vi "Set Power Off Ref.vi"(8 "error in (no error)":errorcluster, 10 "Self Test":refnum<vi>, 11 "Device Under Test In":refnum<class "Device Under Test.lvclass">) -> (0 "error out":errorcluster, 3 "Device Under Test Out":refnum<class "Device Under Test.lvclass">)   [LabVIEW 2021, in "Device Under Test.lvclass"]
uses:
  Device Under Test.lvclass
  C:/Program Files (x86)/National Instruments/LabVIEW 2021/vi.lib/Astemes/Triarc Framework/Process/Process.lvclass
  <vilib>/Astemes/Triarc Framework/Process/Process.lvclass/Process.ctl
  Device Under Test.lvclass/Device Under Test.ctl
  <vilib>/Utility/error.llb/Clear Errors.vi
  <vilib>/Astemes/Triarc Framework/Process/Private/SubVIs/Handle Debug Data.vi
  <vilib>/Utility/High Resolution Relative Seconds.vi
  <vilib>/Utility/error.llb/Error Cluster From Error Code.vi
  <vilib>/Astemes/Triarc Framework/Process/Process.lvclass
  C:/Program Files (x86)/National Instruments/LabVIEW 2021/vi.lib/Astemes/Triarc Framework/View/View.lvclass
  C:/Program Files (x86)/National Instruments/LabVIEW 2021/vi.lib/Astemes/Triarc Framework/Base/Base.lvclass
  C:/Program Files (x86)/National Instruments/LabVIEW 2021/vi.lib/Astemes/Triarc Framework/Error Handler Interface/Error Handler Interface.lvclass
  C:/Program Files (x86)/National Instruments/LabVIEW 2021/vi.lib/Astemes/Triarc Framework/Logging/Logging.lvclass
  C:/Git/astemes-triarc-examples/Thermal Chamber/Device Under Test/Device Under Test.lvclass
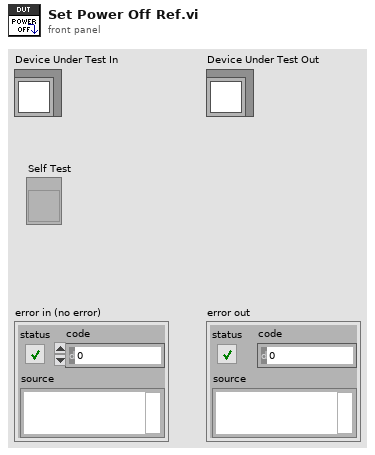
[diagram p1: front panel]
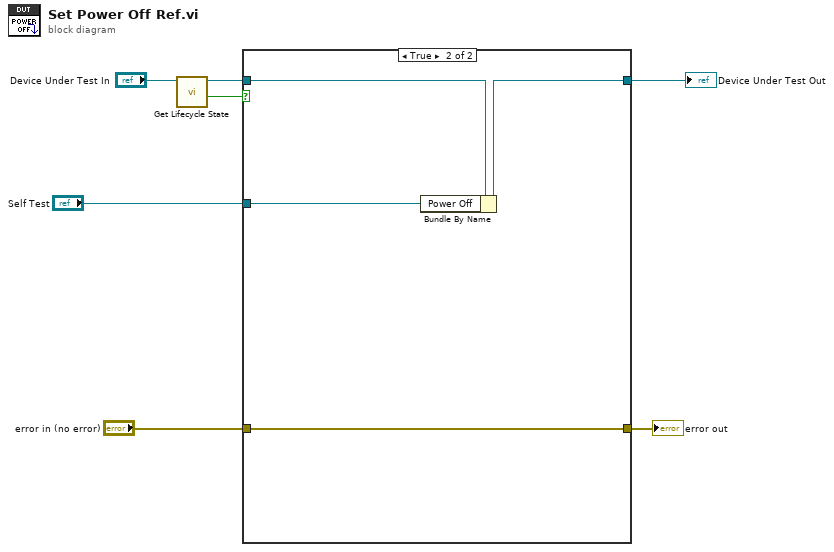
[diagram p0: block diagram]
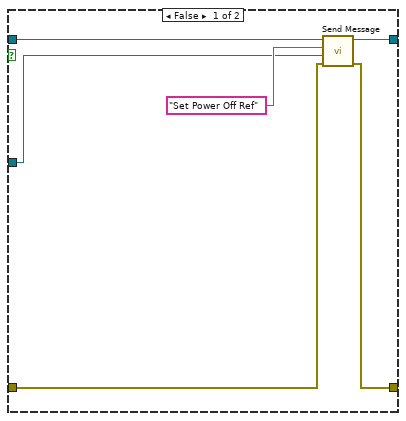
[diagram p2: hidden frame]
diagram:
  n1 = call <vilib>:"Get Lifecycle State.vi"("Process In"="Device Under Test In") -> ("In Process Loop?"=w3:bool, "Process Out"=w6:refnum<class "Device Under Test.lvclass">)  [unwired: 7 in, 2 out]
  n2 = case shown="True" w3 {
    tunnel: w6 -> [w13 w17]
    tunnel: [w12 w15] -> w5
    tunnel: "error in (no error)" -> [w9 w16]
    tunnel: [w10 w16] -> w4
    tunnel: "Self Test" -> [w8 w14]
    frame False {
      n3 = call <vilib>:"Send Message.vi"("error in (no error)"=w9, "Message Data"=w8, "Message"="Set Power Off Ref" ("API Message"), "Process In"=w13) -> ("error out"=w10:errorcluster, "Process Out"=w12:refnum<class "Device Under Test.lvclass">)  [unwired: 6 in]
    }
    frame True {
      n4 = Bundle By Name(cluster=w17, "Power Off"=w14) -> (w15:refnum<class "Device Under Test.lvclass">)
    }
  }
  "error out" <- w4
  "Device Under Test Out" <- w5
